vi "Head Worker Added MHLC.vi"(8 "error in (no error)":errorcluster, 10 "Data in":variant, 11 "Debug Server in":refnum<class "Debug Server.lvclass">) -> (0 "error out":errorcluster, 3 "Debug Server out":refnum<class "Debug Server.lvclass">)   [LabVIEW 2017, in "Debug Server.lvclass"]
doc: "A new Head Worker has been added to the Application Manager. Check if there is already a Message Log for this application. If yes, then tell the TCP Server that the Message Log is ready."
uses:
  Debug Server.lvclass
  C:/Program Files (x86)/National Instruments/LabVIEW 2017/vi.lib/addons/_Workers/Library/Classes/Worker/Worker.lvclass
  Debug Server.lvclass/Debug Server.ctl
  Debug Server TCP Server and Client/Workers/DS TCP Server/rqp_Message Log Ready.ctl
  <vilib>/addons/_Workers/Library/Classes/Message Queue/Message Queue.lvclass
  Common VIs/Message Log ID.ctl
  Common VIs/DC_UID.ctl
  <vilib>/addons/_Workers/Library/Classes/Worker/Worker.lvclass/Worker.ctl
  Message Log/Message Log.lvclass
  Application Manager/Application Manager.lvclass
  Debug Server TCP Server and Client/Workers/DS TCP Server/DS TCP Server.lvclass
  <vilib>/addons/_Workers/Library/Classes/Worker/Worker.lvclass
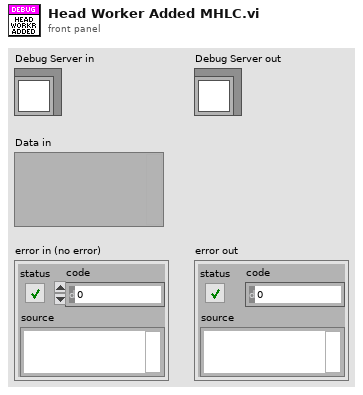
[diagram p1: front panel]
types:
  T1 = typedef "Application Manager.lvclass/rsp_New Head Worker Added.ctl" = cluster{"Head Worker ID":string, "IP Address":string, "DC_UID":T2}
  T2 = typedef "DC_UID.ctl" = string
  T3 = typedef "Debug Server.lvclass/Dynamic Message Log Data.ctl" = cluster{"Message Log":refnum<class "Message Log.lvclass">, "DC_UID":T2, "Message Log ID":T4}
  T4 = typedef "Message Log ID.ctl" = cluster{"Head Worker ID":string, "IP Address":string}
  T5 = typedef "DS TCP Server.lvlib/DS TCP Server.lvclass/rqp_Message Log Ready.ctl" = cluster{"Message Log Q":refnum<class "Message Queue.lvclass">, "Message Log ID":T4, "DC_UID":T2}
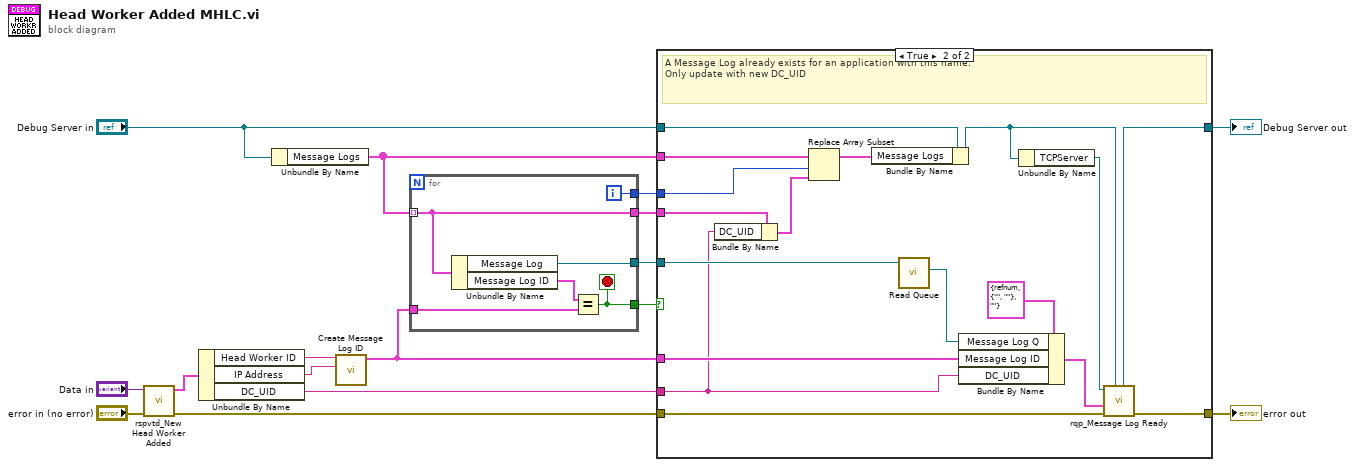
[diagram p0: block diagram]
diagram:
  n1 = call "rspvtd_New Head Worker Added.vi"("error in"="error in (no error)", "Data in"="Data in") -> ("error out"=w11:errorcluster, "Data out"=w6:T1)  [unwired: 8 in]
  n2 = Unbundle By Name(w6) -> ("Head Worker ID"=w7:string, "IP Address"=w8:string, "DC_UID"=w16:T2)
  n3 = Unbundle By Name("Debug Server in") -> ("Message Logs"=w1:T3[])
  n4 = call "Create Message Log ID.vi"("IP Address"=w8, "Head Worker WID"=w7) -> ("Message Log ID"=w15:T4)  [unwired: 9 in]
  n5 = for {
    tunnel: w1 -> [w17] mode=indexing
    tunnel: w15 -> [w21]
    tunnel: [w20] -> w13
    tunnel: [w19] -> w14
    tunnel: [w18] -> w3
    tunnel: [w17] -> w2
    i -> [w18]
    stop <- w20 stop-if-true
    n6 = Unbundle By Name(w17) -> ("Message Log"=w19:refnum<class "Message Log.lvclass">, "Message Log ID"=w22:T4)
    n7 = Equal?(x=w22, y=w21) -> (x = y?=w20:bool)
  }
  n8 = case shown="True" w13 {
    tunnel: "Debug Server in" -> [w24 w38]
    tunnel: [w24 w39] -> w10
    tunnel: w11 -> [w23 w41]
    tunnel: [w23 w40] -> w12
    tunnel: w14 -> [_ w35]
    tunnel: w15 -> [_ w32]
    tunnel: w16 -> [_ w29]
    tunnel: w3 -> [_ w26]
    tunnel: w2 -> [_ w30]
    tunnel: w1 -> [_ w28]
    frame False {
      # "No Message Log exists for this application.\nNothing to do."
    }
    frame True {
      # "A Message Log already exists for an application with this name.\nOnly update with new DC_UID"
      n9 = Bundle By Name(cluster=w30, "DC_UID"=w29) -> (w27:T3)
      n10 = Replace Array Subset(array=w28, new element=w27, index=w26) -> (w25:T3[])
      n11 = Bundle By Name(cluster=w38, "Message Logs"=w25) -> (w31:refnum<class "Debug Server.lvclass">)
      n12 = call <vilib>:"Read Queue.vi"("Worker_"=w35) -> ("Message Queue out"=w34:refnum<class "Message Queue.lvclass">)  [unwired: 9 in, 1 out]
      n13 = Bundle By Name(cluster=T5 {"Message Log Q"=refnum, "Message Log ID"={"Head Worker ID"="", "IP Address"=""}, "DC_UID"=""} ("Data in"), "Message Log Q"=w34, "Message Log ID"=w32, "DC_UID"=w29) -> (w33:T5)
      n14 = Unbundle By Name(w31) -> ("TCPServer"=w37:refnum<class "DS TCP Server.lvclass">)
      n15 = call "rqp_Message Log Ready.vi"("Caller in"=w31, "error in"=w41, "Data in"=w33, "DS TCP Server in"=w37) -> ("error out"=w40:errorcluster, "dup Caller out"=w39:refnum<class "Debug Server.lvclass">)  [unwired: 5 in, 1 out]
    }
  }
  "error out" <- w12
  "Debug Server out" <- w10
